vi "PXDAC4800_GetActiveMemoryRegionXD48.vi"(0 "Handle":u32, 1 "Offset":u32, 2 "Length Byte":u32) -> (3 "Status":i32, 4 "Handle out":u32, 5 "Offset_bytes out":u32, 6 "Playback_bytes out":u32)   [LabVIEW 2016]
uses:
  PXDAC4800.dll
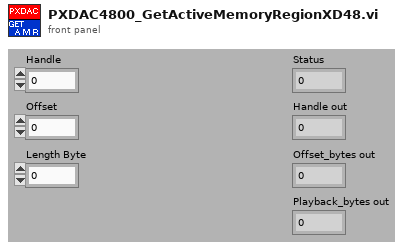
[diagram p1: front panel]
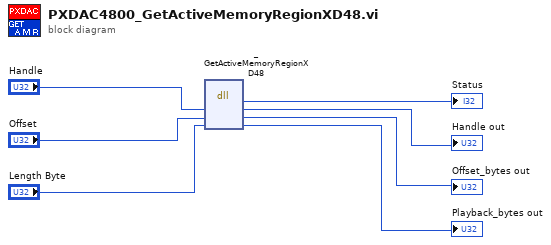
[diagram p0: block diagram]
diagram:
  n1 = dll-call lib="PXDAC4800.dll" fn="_GetActiveMemoryRegionXD48"("Handle"="Handle", "pOffset_bytes"="Offset", "pLength_bytes"="Length Byte") -> (→"Status":i32, "Handle"=→"Handle out":u32, "pOffset_bytes"=→"Offset_bytes out":u32, "pLength_bytes"=→"Playback_bytes out":u32)  [unwired: 3 in, 2 out]
